vi "First_column_names.vi"() -> (0 "Array":string[](array[string]))   [LabVIEW 2020]
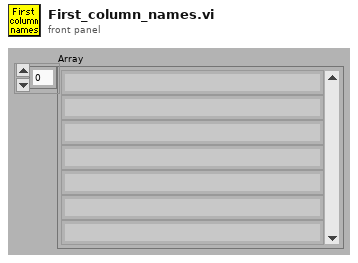
[diagram p1: front panel]
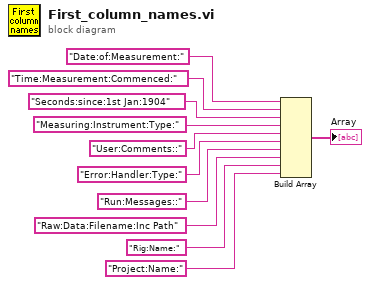
[diagram p0: block diagram]
diagram:
  n1 = Build Array("Date:of:Measurement:", "Time:Measurement:Commenced:", "Seconds:since:1st Jan:1904", "Measuring:Instrument:Type:", "User:Comments::", "Error:Handler:Type:", "Run:Messages::", "Raw:Data:Filename:Inc Path", "Rig:Name:", "Project:Name:") -> (→"Array":string[])
